vi "Score Particles Glenn.vi"(8 "Area Size Limit":i32=444, 9 "Particle Count Limit":i32=10, 10 "Dimensions":cluster{i32, i32}={640, 480}, 11 "Image Refnum in":T1) -> (2 "Scored Particle Info":T2(array[cluster]), 3 "Image Refnum out":T1)   [LabVIEW 2011]
doc: "Score the largest particles in the image to determine how well they match the target attributes. Specifically, calculate how rectangular a particle is, inspect its aspect ratio, and determine if it is hollow (having pixels on around the edges, but off in the large center)."
uses:
  <vilib>/vision/Image Controls.llb/IMAQ Image.ctl
  <vilib>/vision/NI_Vision_Development_Module.lvlib
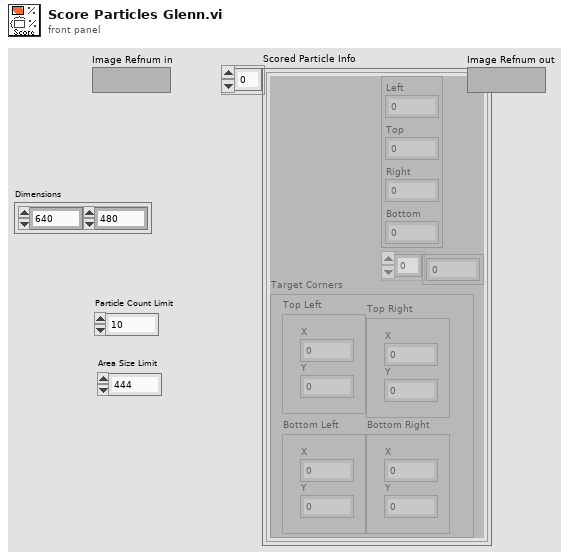
[diagram p1: front panel]
types:
  T1 = typedef "IMAQ Image.ctl" = refnum<image>
  T2 = cluster{cluster{"Left":dbl, "Top":dbl, "Right":dbl, "Bottom":dbl}, dbl[], "Target Corners":cluster{"Bottom Left":cluster{"X":dbl, "Y":dbl}, "Bottom Right":cluster{"X":dbl, "Y":dbl}, "Top Right":cluster{"X":dbl, "Y":dbl}, "Top Left":cluster{"X":dbl, "Y":dbl}}}[]
  T3 = typedef "Particle Parameters" = i32
  T4 = typedef "Image Type" = u32
  T5 = cluster{"Bottom Left":cluster{"X":dbl, "Y":dbl}, "Bottom Right":cluster{"X":dbl, "Y":dbl}, "Top Right":cluster{"X":dbl, "Y":dbl}, "Top Left":cluster{"X":dbl, "Y":dbl}}
  T6 = cluster{"Left":dbl, "Top":dbl, "Right":dbl, "Bottom":dbl}
  T7 = cluster{"Infinite Slope?":bool, "Slope":dbl, "Intercept or X coordinate":dbl}
  T8 = cluster{"[0]":cluster{dbl, dbl}, "[1]":cluster{dbl, dbl}, "[2]":cluster{dbl, dbl}, "[3]":cluster{dbl, dbl}}
  T9 = cluster{cluster{"Left":dbl, "Top":dbl, "Right":dbl, "Bottom":dbl}, dbl[], cluster{"[0]":cluster{dbl, dbl}, "[1]":cluster{dbl, dbl}, "[2]":cluster{dbl, dbl}, "[3]":cluster{dbl, dbl}}}
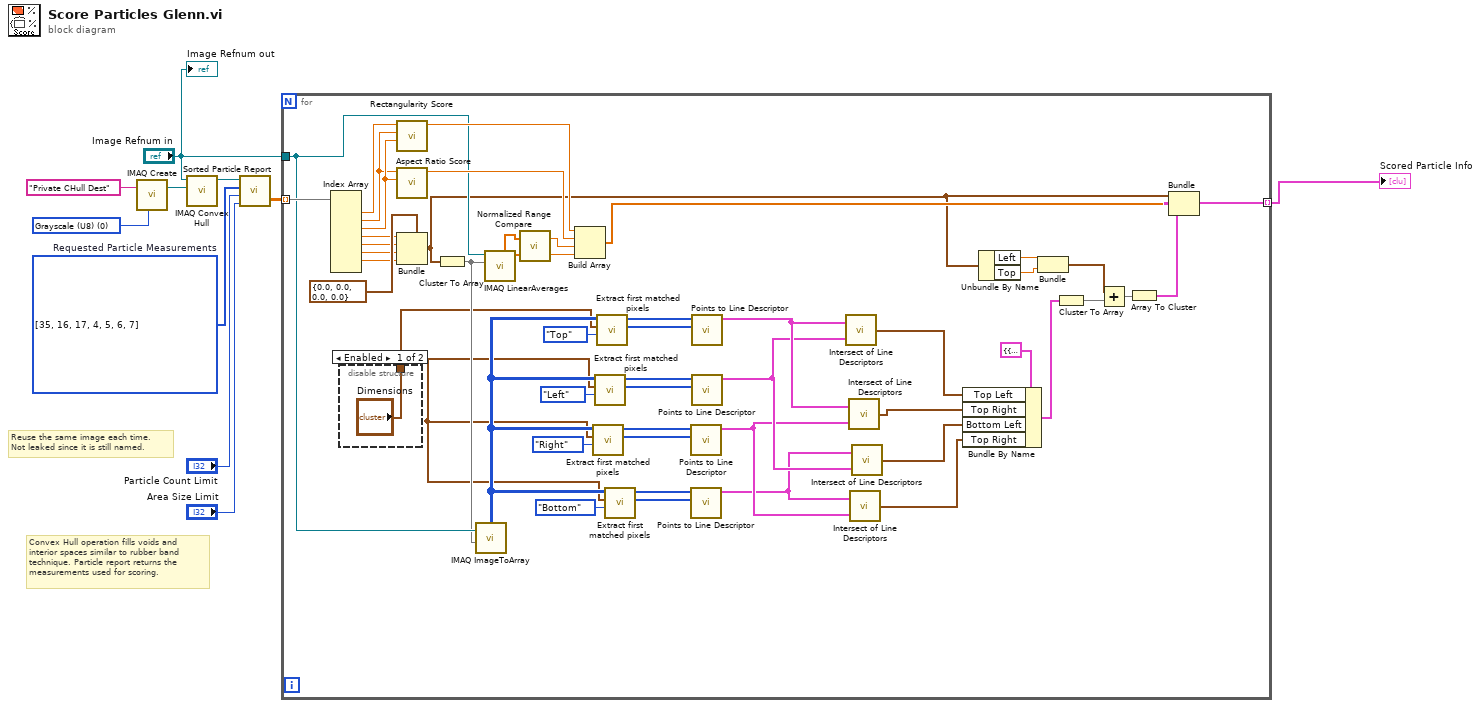
[diagram p0: block diagram]
diagram:
  w2 = T3[] [35, 16, 17, 4, 5, 6, 7] items=["Center of Mass X", "Center of Mass Y", "First Pixel X", "First Pixel Y", "Bounding Rect Left", "Bounding Rect Top", "Bounding Rect Right", "Bounding Rect Bottom", "Max Feret Diameter Start X", "Max Feret Diameter Start Y", "Max Feret Diameter End X", "Max Feret Diameter End Y", "Max Horiz. Segment Length Left", "Max Horiz. Segment Length Right", "Max Horiz. Segment Length Row", "-", "Bounding Rect Width", "Bounding Rect Height", "Bounding Rect Diagonal", "Perimeter", "Convex Hull Perimeter", "Holes' Perimeter", "Max Feret Diameter", "Equivalent Ellipse Major Axis", "Equivalent Ellipse Minor Axis", "Equivalent Ellipse Minor Axis (Feret)", "Equivalent Rect Long Side", "Equivalent Rect Short Side", "Equivalent Rect Diagonal", "Equivalent Rect Short Side (Feret)", "Average Horiz. Segment Length", "Average Vert. Segment Length", "Hydraulic Radius", "Waddel Disk Diameter", "-", "Area", "Holes' Area", "Particle & Holes' Area", "Convex Hull Area", "Image Area", "-", "Number of Holes", "Number of Horiz. Segments", "Number of Vert. Segments", "-", "Orientation", "Max Feret Diameter Orientation", "-", "% Area/Image Area", "% Area/(Particle & Holes' Area)", "Ratio of Equivalent Ellipse Axes", "Ratio of Equivalent Rect Sides", "-", "Elongation Factor", "Compactness Factor", "Heywood Circularity Factor", "Type Factor", "-", "Sum X", "Sum Y", "Sum XX", "Sum XY", "Sum YY", "Sum XXX", "Sum XXY", "Sum XYY", "Sum YYY", "-", "Moment of Inertia XX", "Moment of Inertia XY", "Moment of Inertia YY", "Moment of Inertia XXX", "Moment of Inertia XXY", "Moment of Inertia XYY", "Moment of Inertia YYY", "Norm. Moment of Inertia XX", "Norm. Moment of Inertia XY", "Norm. Moment of Inertia YY", "Norm. Moment of Inertia XXX", "Norm. Moment of Inertia XXY", "Norm. Moment of Inertia XYY", "Norm. Moment of Inertia YYY", "Hu Moment 1", "Hu Moment 2", "Hu Moment 3", "Hu Moment 4", "Hu Moment 5", "Hu Moment 6", "Hu Moment 7"]  # Requested Particle Measurements
  w8 = T4 0 items=["Grayscale (U8)", "Grayscale (I16)", "Grayscale (SGL)", "Complex (CSG)", "RGB (U32)", "HSL (U32)", "RGB (U64)", "Grayscale (U16)"] ("Image Type")
  # "Reuse the same image each time.\nNot leaked since it is still named."
  # "Convex Hull operation fills voids and\ninterior spaces similar to rubber band\ntechnique. Particle report returns the\nmeasurements used for scoring."
  n1 = call "IMAQ Create"("Image Name"="Private CHull Dest", "Image Type"=w8) -> ("New Image"=w7:T1)  [unwired: 2 in, 2 out]
  n2 = call "IMAQ Convex Hull"("Image Dst"=w7, "Image Src"="Image Refnum in") -> ("Image Dst Out"=w5:T1)  [unwired: 2 in, 7 out]
  n3 = call "Sorted Particle Report.vi"("Area Size Limit"="Area Size Limit", "Particle Count Limit"="Particle Count Limit", "Pixel Measurements"=w2, "Image in"=w5) -> ("Sorted Data"=w10:dbl[][])  [unwired: 1 out]
  n4 = for {
    tunnel: [w58] -> w1 mode=indexing
    tunnel: "Image Refnum in" -> [w43]
    tunnel: w10 -> [w50] mode=indexing
    n5 = Index Array(array=w50) -> (element #1=w59:dbl, element #2=w44:dbl, element #3=w45:dbl, element #4=w46:dbl, element #5=w47:dbl, element #6=w48:dbl, element #7=w49:dbl)  [unwired: 8 in, 1 out]
    n6 = disable-structure shown="Enabled" {
      disable-tunnel: ["Dimensions" _] -> w11
      frame Enabled {
      }
      frame Disabled {
      }
    }
    n7 = call "Rectangularity Score.vi"("Height"=w45, "Width"=w44, "Area"=w59) -> ("Score"=w53:dbl)  [unwired: 8 in]
    n8 = call "Aspect Ratio Score.vi"("Height"=w45, "Width"=w44) -> ("Score"=w54:dbl)  [unwired: 9 in]
    n9 = Bundle(cluster=T6 {"Left"=0.0, "Top"=0.0, "Right"=0.0, "Bottom"=0.0}, "Left"=w46, "Top"=w47, "Right"=w48, "Bottom"=w49) -> (w23:T6)
    n10 = Cluster To Array(cluster=w23) -> (array=w42:dbl[])
    n11 = call "IMAQ ImageToArray"("Optional Rectangle"=w42, "Image"=w43) -> ("Image Pixels (U8)"=w40:u8[][])  [unwired: 2 in, 4 out]
    n12 = call "IMAQ LinearAverages"("Optional Rectangle"=w42, "Image Src"=w43) -> ("Y Axis Averages"=w52:sgl[], "X Axis Averages"=w51:sgl[])  [unwired: 2 in, 6 out]
    n13 = call "Normalized Range Compare.vi"("Y Averages"=w52, "X Averages"=w51) -> ("Y Score"=w56:dbl, "X Score"=w55:dbl)
    n14 = Build Array(w53, w54, w55, w56) -> (w57:dbl[])
    n15 = call "Extract first matched pixels.vi"("Side"=enum16{"Top", "Left", "Bottom", "Right"}."Right", "Dimensions"=w11, "Image Pixels (U8)"=w40) -> ("Y out"=w14:i16[], "X out"=w15:i16[])  [unwired: 7 in]
    n16 = call "Extract first matched pixels.vi"("Side"=enum16{"Top", "Left", "Bottom", "Right"}."Left", "Dimensions"=w11, "Image Pixels (U8)"=w40) -> ("Y out"=w16:i16[], "X out"=w17:i16[])  [unwired: 7 in]
    n17 = call "Extract first matched pixels.vi"("Side"=enum16{"Top", "Left", "Bottom", "Right"}."Top", "Dimensions"=w11, "Image Pixels (U8)"=w40) -> ("Y out"=w38:i16[], "X out"=w39:i16[])  [unwired: 7 in]
    n18 = call "Extract first matched pixels.vi"("Side"=enum16{"Top", "Left", "Bottom", "Right"}."Bottom", "Dimensions"=w11, "Image Pixels (U8)"=w40) -> ("Y out"=w18:i16[], "X out"=w19:i16[])  [unwired: 7 in]
    n19 = call "Points to Line Descriptor.vi"("Y"=w14, "X"=w15) -> ("Line out"=w13:T7)  [unwired: 9 in]
    n20 = call "Points to Line Descriptor.vi"("Y"=w18, "X"=w19) -> ("Line out"=w12:T7)  [unwired: 9 in]
    n21 = call "Points to Line Descriptor.vi"("Y"=w38, "X"=w39) -> ("Line out"=w37:T7)  [unwired: 9 in]
    n22 = call "Points to Line Descriptor.vi"("Y"=w16, "X"=w17) -> ("Line out"=w36:T7)  [unwired: 9 in]
    n23 = call "Intersect of Line Descriptors.vi"("Line B"=w36, "Line A"=w37) -> ("Intersect"=w35:cluster{"X":dbl, "Y":dbl})  [unwired: 1 in]
    n24 = call "Intersect of Line Descriptors.vi"("Line B"=w13, "Line A"=w37) -> ("Intersect"=w34:cluster{"X":dbl, "Y":dbl})  [unwired: 1 in]
    n25 = call "Intersect of Line Descriptors.vi"("Line B"=w13, "Line A"=w12) -> ("Intersect"=w32:cluster{"X":dbl, "Y":dbl})  [unwired: 1 in]
    n26 = call "Intersect of Line Descriptors.vi"("Line B"=w36, "Line A"=w12) -> ("Intersect"=w33:cluster{"X":dbl, "Y":dbl})  [unwired: 1 in]
    n27 = Bundle By Name(cluster=T5 {"Bottom Left"={"X"=0.0, "Y"=0.0}, "Bottom Right"={"X"=0.0, "Y"=0.0}, "Top Right"={"X"=0.0, "Y"=0.0}, "Top Left"={"X"=0.0, "Y"=0.0}} ("Target Corners"), "Top Left"=w35, "Top Right"=w34, "Bottom Left"=w33, "Top Right"=w32) -> (w29:T5)
    n28 = Unbundle By Name(w23) -> ("Left"=w31:dbl, "Top"=w30:dbl)
    n29 = Bundle("Left"=w31, "Top"=w30) -> (w24:cluster{"Left":dbl, "Top":dbl})  [unwired: 1 in]
    n30 = Cluster To Array(cluster=w29) -> (array=w25:cluster{"X":dbl, "Y":dbl}[])
    n31 = Add(x=w24, y=w25) -> (x+y=w26:cluster{dbl, dbl}[])
    n32 = Array To Cluster(array=w26) -> (cluster=w27:T8)
    n33 = Bundle(w23, w57, w27) -> (w58:T9)  [unwired: 1 in]
  }
  "Scored Particle Info" <- w1
  "Image Refnum out" <- "Image Refnum in"
